vi "LVH5TGetLVType.vi"(7 "Don't use cache":bool, 8 "error in (no error)":errorcluster, 9 "Type":enum16{"File", "Memory"}(ring)=enum."Memory", 10 "Name":string, 11 "HDF5 Type Ref":T1) -> (0 "error out":errorcluster, 1 "Type String":i16[](array[numeric]) format="%.0x", 2 "Data Type":variant, 3 "HDF5 Type Ref out":T1, 4 "Description":string)   [LabVIEW 2017]
doc: "Creates a variant containg a LabVIEW datatype which corresponds to an HDF5 datatype."
uses:
  <vilib>/UPVI/lvhdf5/library.llb/HDF5 Ref.ctl
  <vilib>/UPVI/lvhdf5/datatype.llb/private/LVTypeElement.ctl
  <vilib>/Utility/VariantDataType/UnitInfo.ctl
  <vilib>/Utility/VariantDataType/UnitType.ctl
  <vilib>/UPVI/lvhdf5/error.llb/LVH5EMajorID.ctl
  <vilib>/UPVI/lvhdf5/error.llb/LVH5EMinorID.ctl
  <userlib>/_OpenG.lib/lvdata/lvdata.llb/Type Descriptor Enumeration__ogtk.ctl
  <vilib>/UPVI/lvhdf5/datatype.llb/H5T_sign_t.ctl
  <vilib>/UPVI/lvhdf5/datatype.llb/LVH5ClassID.ctl
  <vilib>/UPVI/lvhdf5/reference.llb/H5R Object Ref.ctl
  <vilib>/UPVI/lvhdf5/reference.llb/H5R Dataset Region Ref.ctl
  <vilib>/UPVI/lvhdf5/error.llb/H5Epush_enum_enum.vi
  <vilib>/Utility/VariantDataType/VariantType.lvlib
panel:
  # "LVHDF5 Toolkit\nCopyright (c) 2005-2013 by Jason D. Sommerville\nCopyright (c) 2014 by UPVI, LLC.\n\nThis use and distribution of this file is governed by the terms found in \nLICENSE.txt distributed with this toolkit and installed at\n <user.lib>\\_lvhdf5\\LICENSE.txt"
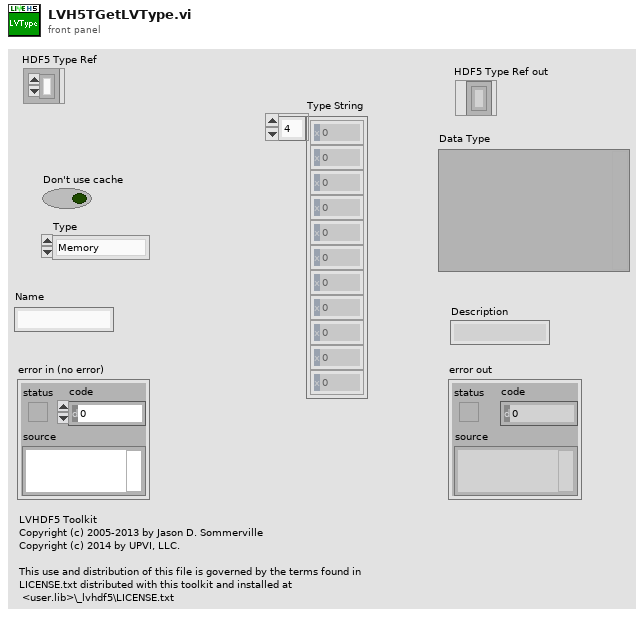
[diagram p1: front panel]
types:
  T1 = typedef "HDF5 Ref.ctl" = refnum<k1>
  T2 = enum16{"find by lvtype", "find by h5type", "index", "push", "pop", "delete last", "dequeue", "delete all"}
  T3 = typedef "LVTypeElement.ctl" = cluster{"Name":string, "TD":i16[], "Type Ref":T1, "Description":string, "Unit String":string, "Units":T4[], "Status":cluster{"MustCommit":bool, "IsCommitted":bool}}
  T4 = typedef "VariantType.lvlib/UnitInfo.ctl" = cluster{"UnitType":T5, "Exponent":i16}
  T5 = typedef "VariantType.lvlib/UnitType.ctl" = enum16{"Radians", "Steradians", "Seconds", "Meters", "Kilograms", "Amperes", "Kelvins", "Moles", "Candelas", "InvalidUnit"}
  T6 = typedef "LVH5EMinorID.ctl" = string
  T7 = typedef "LVH5EMajorID.ctl" = string
  T8 = typedef "Type Descriptor Enumeration__ogtk.ctl" = enum8{"<Null>", "I8", "I16", "I32", "I64", "U8", "U16", "U32", "U64", "SGL", "DBL", "EXT", "CSG", "CDB", "CXT", "0x0F", "0x10", "0x11", "0x12", "0x13", "0x14", "Enum U8", "Enum U16", "Enum U32", "Enum U64", "SGL PQ", "DBL PQ", "EXT PQ", "CSG PQ", "CDB PQ", "CXT PQ", "0x1F", "0x20", "Boolean", "0x22", "0x23", "0x24", "0x25", "0x26", "0x27", "0x28", "0x29", "0x2A", "0x2B", "0x2C", "0x2D", "0x2E", "0x2F", "String", "0x31", "Path", "Pict", "0x34", "0x35", "0x36", "DAQ", "0x38", "0x39", "0x3A", "0x3B", "0x3C", "0x3D", "0x3E", "0x3F", "Array", "0x41", "0x42", "0x43", "0x44", "0x45", "0x46", "0x47", "0x48", "0x49", "0x4A", "0x4B", "0x4C", "0x4D", "0x4E", "0x4F", "Cluster", "0x51", "0x52", "Variant", "Waveform", "0x55", "0x56", "0x57", "0x58", "0x59", "0x5A", "0x5B", "0x5C", "0x5D", "0x5E", "0x5F", "0x60", "0x61", "0x62", "0x63", "0x64", "0x65", "0x66", "0x67", "0x68", "0x69", "0x6A", "0x6B", "0x6C", "0x6D", "0x6E", "0x6F", "Refnum"}
  T9 = typedef "LVH5ClassID.ctl" = enum32{"H5T_IEEE_F32BE", "H5T_IEEE_F32LE", "H5T_IEEE_F64BE", "H5T_IEEE_F64LE", "H5T_STD_I8BE", "H5T_STD_I8LE", "H5T_STD_I16BE", "H5T_STD_I16LE", "H5T_STD_I32BE", "H5T_STD_I32LE", "H5T_STD_I64BE", "H5T_STD_I64LE", "H5T_STD_U8BE", "H5T_STD_U8LE", "H5T_STD_U16BE", "H5T_STD_U16LE", "H5T_STD_U32BE", "H5T_STD_U32LE", "H5T_STD_U64BE", "H5T_STD_U64LE", "H5T_STD_B8BE", "H5T_STD_B8LE", "H5T_STD_B16BE", "H5T_STD_B16LE", "H5T_STD_B32BE", "H5T_STD_B32LE", "H5T_STD_B64BE", "H5T_STD_B64LE", "H5T_STD_REF_OBJ", "H5T_STD_REF_DSETREG", "H5T_UNIX_D32BE", "H5T_UNIX_D32LE", "H5T_UNIX_D64BE", "H5T_UNIX_D64LE", "H5T_C_S1", "H5T_FORTRAN_S1", "H5T_INTEL_I8", "H5T_INTEL_I16", "H5T_INTEL_I32", "H5T_INTEL_I64", "H5T_INTEL_U8", "H5T_INTEL_U16", "H5T_INTEL_U32", "H5T_INTEL_U64", "H5T_INTEL_B8", "H5T_INTEL_B16", "H5T_INTEL_B32", "H5T_INTEL_B64", "H5T_INTEL_F32", "H5T_INTEL_F64", "H5T_ALPHA_I8", "H5T_ALPHA_I16", "H5T_ALPHA_I32", "H5T_ALPHA_I64", "H5T_ALPHA_U8", "H5T_ALPHA_U16", "H5T_ALPHA_U32", "H5T_ALPHA_U64", "H5T_ALPHA_B8", "H5T_ALPHA_B16", "H5T_ALPHA_B32", "H5T_ALPHA_B64", "H5T_ALPHA_F32", "H5T_ALPHA_F64", "H5T_MIPS_I8", "H5T_MIPS_I16", "H5T_MIPS_I32", "H5T_MIPS_I64", "H5T_MIPS_U8", "H5T_MIPS_U16", "H5T_MIPS_U32", "H5T_MIPS_U64", "H5T_MIPS_B8", "H5T_MIPS_B16", "H5T_MIPS_B32", "H5T_MIPS_B64", "H5T_MIPS_F32", "H5T_MIPS_F64", "H5T_NATIVE_CHAR", "H5T_NATIVE_SCHAR", "H5T_NATIVE_UCHAR", "H5T_NATIVE_SHORT", "H5T_NATIVE_USHORT", "H5T_NATIVE_INT", "H5T_NATIVE_UINT", "H5T_NATIVE_LONG", "H5T_NATIVE_ULONG", "H5T_NATIVE_LLONG", "H5T_NATIVE_ULLONG", "H5T_NATIVE_FLOAT", "H5T_NATIVE_DOUBLE", "H5T_NATIVE_LDOUBLE", "H5T_NATIVE_B8", "H5T_NATIVE_B16", "H5T_NATIVE_B32", "H5T_NATIVE_B64", "H5T_NATIVE_OPAQUE", "H5T_NATIVE_HADDR", "H5T_NATIVE_HSIZE", "H5T_NATIVE_HSSIZE", "H5T_NATIVE_HERR", "H5T_NATIVE_HBOOL", "H5T_NATIVE_INT8", "H5T_NATIVE_UINT8", "H5T_NATIVE_INT_LEAST8", "H5T_NATIVE_UINT_LEAST8", "H5T_NATIVE_INT_FAST8", "H5T_NATIVE_UINT_FAST8", "H5T_NATIVE_INT16", "H5T_NATIVE_UINT16", "H5T_NATIVE_INT_LEAST16", "H5T_NATIVE_UINT_LEAST16", "H5T_NATIVE_INT_FAST16", "H5T_NATIVE_UINT_FAST16", "H5T_NATIVE_INT32", "H5T_NATIVE_UINT32", "H5T_NATIVE_INT_LEAST32", "H5T_NATIVE_UINT_LEAST32", "H5T_NATIVE_INT_FAST32", "H5T_NATIVE_UINT_FAST32", "H5T_NATIVE_INT64", "H5T_NATIVE_UINT64", "H5T_NATIVE_INT_LEAST64", "H5T_NATIVE_UINT_LEAST64", "H5T_NATIVE_INT_FAST64"}
  T10 = typedef "H5T_sign_t.ctl" = i32
  T11 = typedef "H5R Object Ref.ctl" = refnum<k1>
  T12 = typedef "H5R Dataset Region Ref.ctl" = refnum<k1>
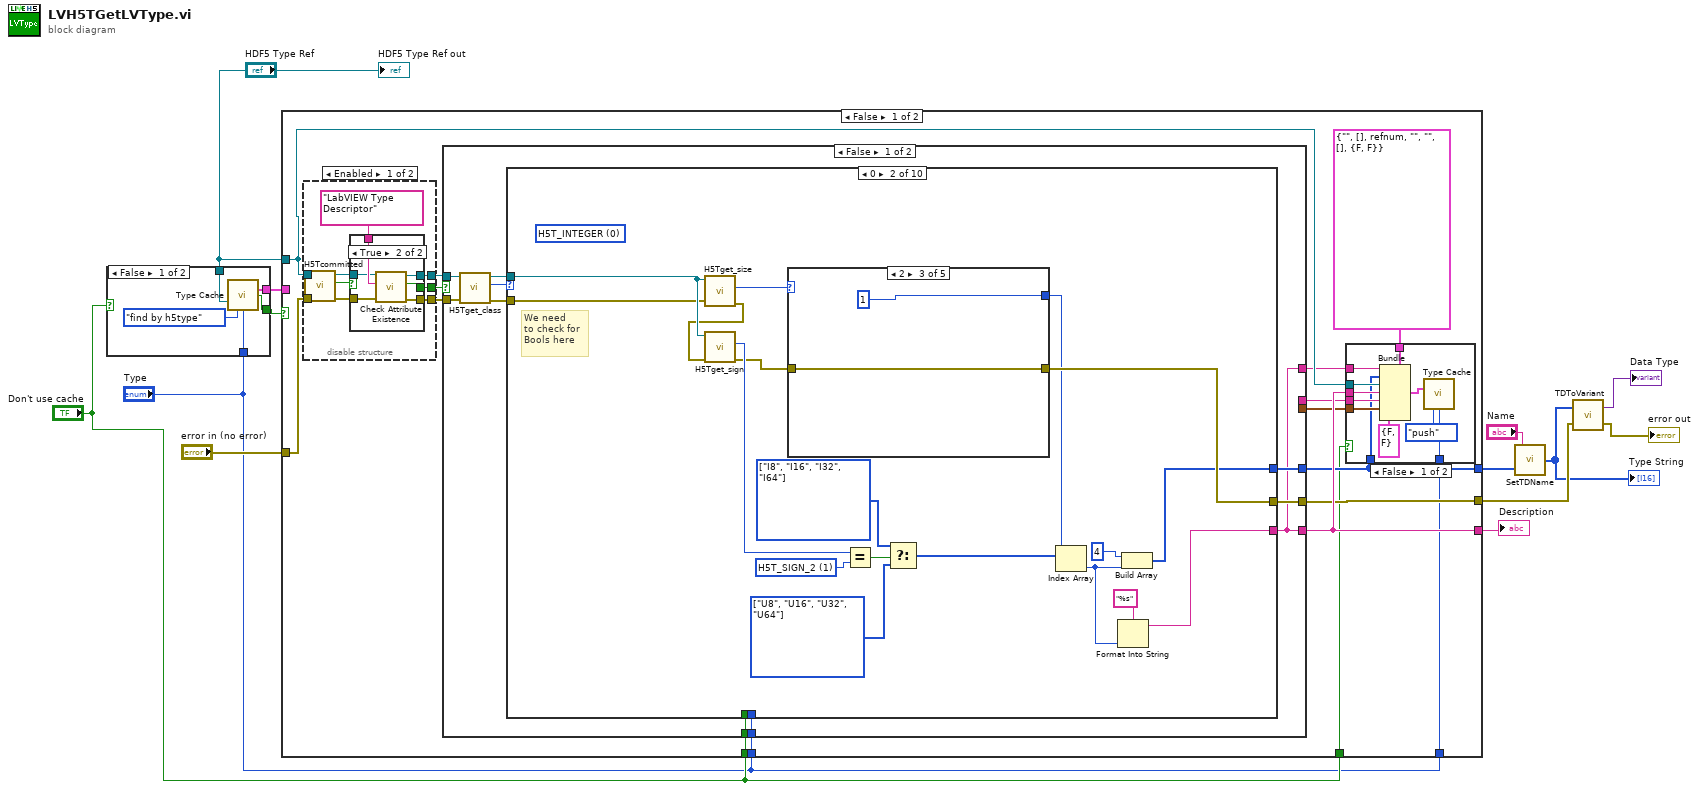
[diagram p0: block diagram]
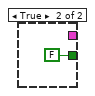
[diagram p2: hidden frame]
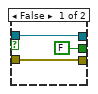
[diagram p4: hidden frame]
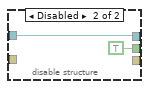
[diagram p5: hidden frame]
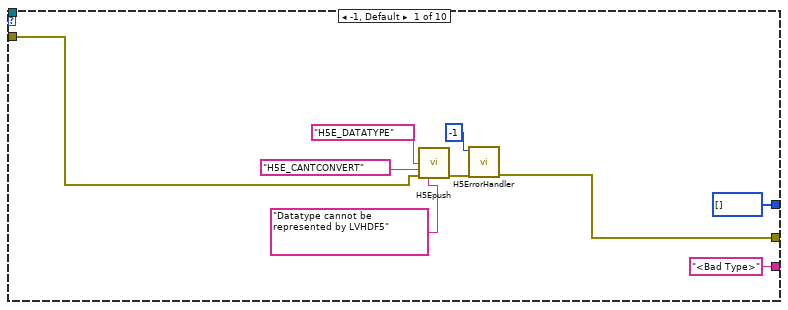
[diagram p6: hidden frame]
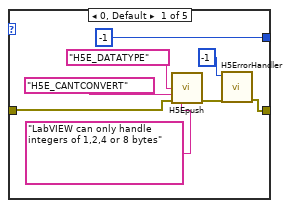
[diagram p7: hidden frame]
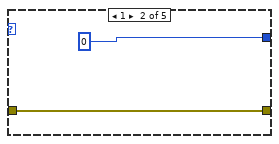
[diagram p8: hidden frame]
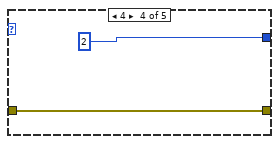
[diagram p9: hidden frame]
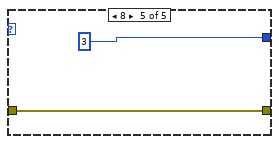
[diagram p10: hidden frame]
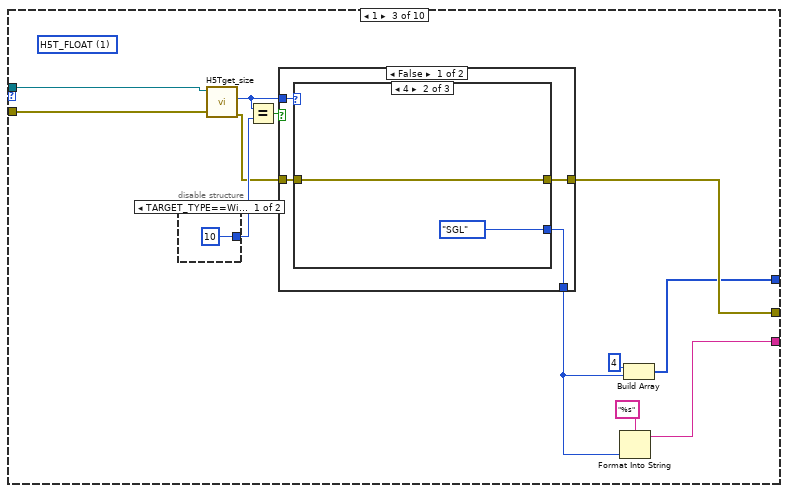
[diagram p11: hidden frame]
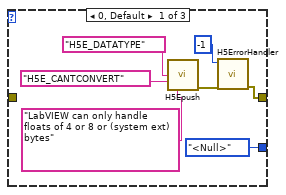
[diagram p12: hidden frame]
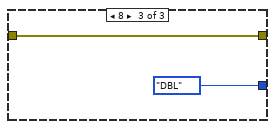
[diagram p13: hidden frame]
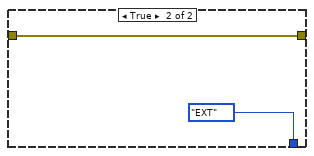
[diagram p14: hidden frame]
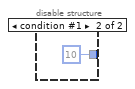
[diagram p15: hidden frame]
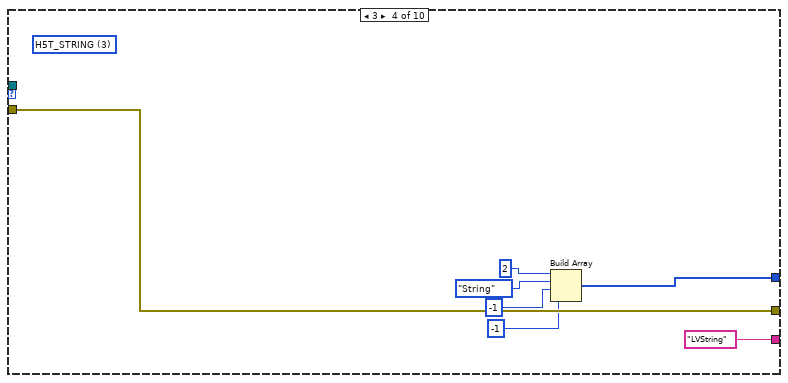
[diagram p16: hidden frame]
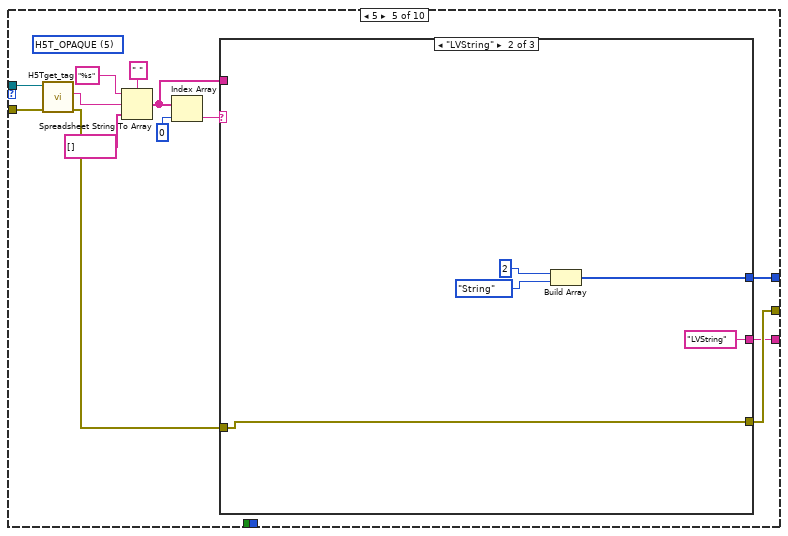
[diagram p17: hidden frame]
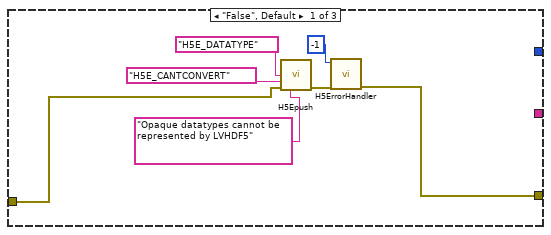
[diagram p18: hidden frame]
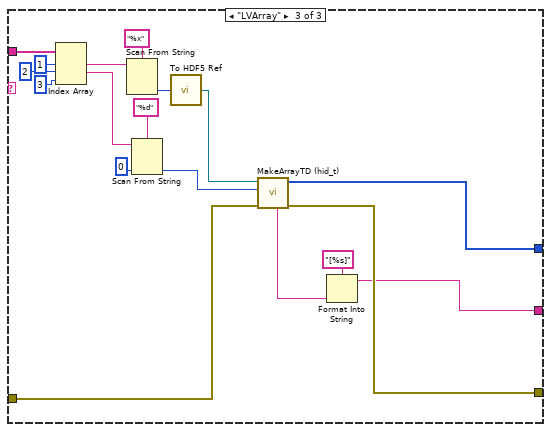
[diagram p19: hidden frame]
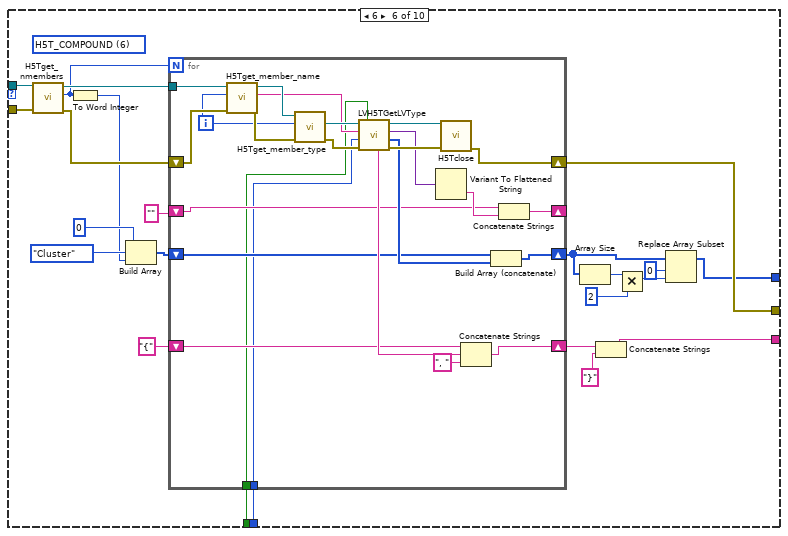
[diagram p20: hidden frame]
diagram:
  n1 = case shown="False" "Don't use cache" {
    tunnel: "HDF5 Type Ref" -> [w18 _]
    tunnel: [w17 _] -> w12
    tunnel: [w16 FALSE ("Found?")] -> w11
    tunnel: "Type" -> [w14 _]
    frame False {
      n2 = call <vilib>:"Type Cache.vi"("H5Type (for find)"=w18, "operation"=T2."find by h5type", "Type"=w14) -> ("LVTypeElement out"=w17:T3, "Found?"=w16:bool)  [unwired: 9 in, 2 out]
    }
    frame True {
    }
  }
  n3 = case shown="False" w11 {
    tunnel: "error in (no error)" -> [w32 w562]
    tunnel: [w24 w561] -> w8
    tunnel: "HDF5 Type Ref" -> [w30 _]
    tunnel: w12 -> [_ w564]
    tunnel: [w28 w563] -> w10
    tunnel: [w25 w562] -> w7
    tunnel: "Don't use cache" -> [w23 _]
    tunnel: "Type" -> [w22 _]
    tunnel: "Don't use cache" -> [w21 _]
    tunnel: "Type" -> [w20 _]
    frame False {
      n4 = disable-structure shown="Enabled" {
        disable-tunnel: [w55 _] -> w35
        disable-tunnel: [w54 TRUE ("Exists")] -> w34
        disable-tunnel: [w52 w66] -> w33
        disable-tunnel: w32 -> [w50 _]
        disable-tunnel: w30 -> [w47 w66]
        frame Enabled {
          n5 = call <vilib>:"H5Tcommitted.vi"("error in (no error)"=w50, "HDF5Type  Ref"=w47) -> ("error out"=w49:errorcluster, "Committed"=w48:bool, "HDF5 Type Ref out"=w51:T1)  [unwired: 5 in]
          n6 = case shown="True" w48 {
            tunnel: [w56 w64] -> w55
            tunnel: [FALSE ("Exists") w63] -> w54
            tunnel: "LabVIEW Type Descriptor" ("name") -> [_ w62]
            tunnel: [w58 w61] -> w52
            tunnel: w51 -> [w58 w60]
            tunnel: w49 -> [w56 w59]
            frame False {
            }
            frame True {
              n7 = call <vilib>:"Check Attribute Existence.vi"("error in (no error)"=w59, "name"=w62, "HDF5 Ref"=w60) -> ("error out"=w64:errorcluster, "Exists"=w63:bool, "HDF5 Ref out"=w61:T1)  [unwired: 4 in]
            }
          }
        }
        frame Disabled {
        }
      }
      n8 = case shown="False" w34 {
        tunnel: [w69 w552] -> w28
        tunnel: [w73 w560] -> w24
        tunnel: [w72 w557] -> w25
        tunnel: w33 -> [w71 w556]
        tunnel: w35 -> [w70 w555]
        tunnel: [w69 w547] -> w29
        tunnel: [_ w559] -> w27
        tunnel: [_ w558] -> w26
        tunnel: w21 -> [w68 _]
        tunnel: w20 -> [w67 _]
        frame False {
          n9 = call <vilib>:"H5Tget_class.vi"("error in (no error)"=w70, "HDF5 Type Ref"=w71) -> ("error out"=w74:errorcluster, "class"=w76:i32, "HDF5 Type Ref out"=w75:T1)  [unwired: 5 in]
          n10 = case shown="0" w76 {
            tunnel: w75 -> [_ w103 w131 _ w170 w223 w255 w300 w529 w544]
            tunnel: w74 -> [w79 w102 w130 w153 w169 w222 w258 w298 w528 w543]
            tunnel: [i16[] [] ("td") w100 w128 w157 w163 w219 w250 w296 w531 w546] -> w73
            tunnel: [w80 w101 w129 w153 w159 w220 w248 w295 w527 w542] -> w72
            tunnel: ["<Bad Type>" w99 w127 "LVString" w158 w221 w249 w294 w530 w545] -> w69
            tunnel: w68 -> [_ _ _ _ _ w201 _ _ w520 w533]
            tunnel: w67 -> [_ _ _ _ _ w202 _ _ w519 w532]
            frame -1, Default {
              n11 = call-poly <vilib>:"H5Epush.vi"("major_id"=T7 "H5E_DATATYPE", "minor_id"=T6 "H5E_CANTCONVERT", "error in (no error)"=w79, "msg"="Datatype cannot be represented by LVHDF5") -> ("error out"=w81:errorcluster)  [unwired: 10 in, 1 out]
              n12 = call <vilib>:"H5ErrorHandler.vi"("error in (no error)"=w81, "herr_t"=-1) -> ("error out"=w80:errorcluster)  [unwired: 3 in, 4 out]
            }
            frame 0 {
              w97 = T10 1 items=["H5T_SIGN_ERROR"=-1, "H5T_SIGN_NONE"=0, "H5T_SIGN_2"=1] ("Sign")
              w93 = T8[] [enum."U8", enum."U16", enum."U32", enum."U64"] items=["<Null>", "I8", "I16", "I32", "I64", "U8", "U16", "U32", "U64", "SGL", "DBL", "EXT", "CSG", "CDB", "CXT", "0x0F", "0x10", "0x11", "0x12", "0x13", "0x14", "Enum U8", "Enum U16", "Enum U32", "Enum U64", "SGL PQ", "DBL PQ", "EXT PQ", "CSG PQ", "CDB PQ", "CXT PQ", "0x1F", "0x20", "Boolean", "0x22", "0x23", "0x24", "0x25", "0x26", "0x27", "0x28", "0x29", "0x2A", "0x2B", "0x2C", "0x2D", "0x2E", "0x2F", "String", "0x31", "Path", "Pict", "0x34", "0x35", "0x36", "DAQ", "0x38", "0x39", "0x3A", "0x3B", "0x3C", "0x3D", "0x3E", "0x3F", "Array", "0x41", "0x42", "0x43", "0x44", "0x45", "0x46", "0x47", "0x48", "0x49", "0x4A", "0x4B", "0x4C", "0x4D", "0x4E", "0x4F", "Cluster", "0x51", "0x52", "Variant", "Waveform", "0x55", "0x56", "0x57", "0x58", "0x59", "0x5A", "0x5B", "0x5C", "0x5D", "0x5E", "0x5F", "0x60", "0x61", "0x62", "0x63", "0x64", "0x65", "0x66", "0x67", "0x68", "0x69", "0x6A", "0x6B", "0x6C", "0x6D", "0x6E", "0x6F", "Refnum"]
              w94 = T8[] [enum."I8", enum."I16", enum."I32", enum."I64"] items=["<Null>", "I8", "I16", "I32", "I64", "U8", "U16", "U32", "U64", "SGL", "DBL", "EXT", "CSG", "CDB", "CXT", "0x0F", "0x10", "0x11", "0x12", "0x13", "0x14", "Enum U8", "Enum U16", "Enum U32", "Enum U64", "SGL PQ", "DBL PQ", "EXT PQ", "CSG PQ", "CDB PQ", "CXT PQ", "0x1F", "0x20", "Boolean", "0x22", "0x23", "0x24", "0x25", "0x26", "0x27", "0x28", "0x29", "0x2A", "0x2B", "0x2C", "0x2D", "0x2E", "0x2F", "String", "0x31", "Path", "Pict", "0x34", "0x35", "0x36", "DAQ", "0x38", "0x39", "0x3A", "0x3B", "0x3C", "0x3D", "0x3E", "0x3F", "Array", "0x41", "0x42", "0x43", "0x44", "0x45", "0x46", "0x47", "0x48", "0x49", "0x4A", "0x4B", "0x4C", "0x4D", "0x4E", "0x4F", "Cluster", "0x51", "0x52", "Variant", "Waveform", "0x55", "0x56", "0x57", "0x58", "0x59", "0x5A", "0x5B", "0x5C", "0x5D", "0x5E", "0x5F", "0x60", "0x61", "0x62", "0x63", "0x64", "0x65", "0x66", "0x67", "0x68", "0x69", "0x6A", "0x6B", "0x6C", "0x6D", "0x6E", "0x6F", "Refnum"]
              (unwired) 0 items=["H5T_NO_CLASS"=-1, "H5T_INTEGER"=0, "H5T_FLOAT"=1, "H5T_TIME"=2, "H5T_STRING"=3, "H5T_BITFIELD"=4, "H5T_OPAQUE"=5, "H5T_COMPOUND"=6, "H5T_REFERENCE"=7, "H5T_ENUM"=8, "H5T_VLEN"=9, "H5T_ARRAY"=10] ("class")
              # "We need\nto check for\nBools here"
              n13 = call <vilib>:"H5Tget_size.vi"("error in (no error)"=w102, "HDF5 Type Ref"=w103) -> ("error out"=w98:errorcluster, "Size"=w86:u32)  [unwired: 5 in, 1 out]
              n14 = call <vilib>:"H5Tget_sign.vi"("error in (no error)"=w98, "HDF5 Ref"=w103) -> ("error out"=w90:errorcluster, "Sign"=w96:T10)  [unwired: 5 in, 1 out]
              n15 = case shown="2" w86 {
                tunnel: [-1 0 1 2 3] -> w91
                tunnel: w90 -> [w105 w112 w114 w116 w118]
                tunnel: [w104 w112 w114 w116 w118] -> w101
                frame 0, Default {
                  n16 = call-poly <vilib>:"H5Epush.vi"("major_id"=T7 "H5E_DATATYPE", "minor_id"=T6 "H5E_CANTCONVERT", "error in (no error)"=w105, "msg"="LabVIEW can only handle integers of 1,2,4 or 8 bytes") -> ("error out"=w106:errorcluster)  [unwired: 10 in, 1 out]
                  n17 = call <vilib>:"H5ErrorHandler.vi"("error in (no error)"=w106, "herr_t"=-1) -> ("error out"=w104:errorcluster)  [unwired: 3 in, 4 out]
                }
                frame 1 {
                }
                frame 2 {
                }
                frame 4 {
                }
                frame 8 {
                }
              }
              n18 = Equal?(x=w96, y=w97) -> (x = y?=w95:bool)
              n19 = Select(t=w94, s=w95, f=w93) -> (s? t:f=w92:T8[])
              n20 = Index Array(array=w92, index=w91) -> (element=w88:T8)
              n21 = Format Into String(format string="%s", w88) -> (resulting string=w99:string)  [unwired: 2 in, 1 out]
              n22 = Build Array(i16 4, w88) -> (w100:i16[])
            }
            frame 1 {
              (unwired) 1 items=["H5T_NO_CLASS"=-1, "H5T_INTEGER"=0, "H5T_FLOAT"=1, "H5T_TIME"=2, "H5T_STRING"=3, "H5T_BITFIELD"=4, "H5T_OPAQUE"=5, "H5T_COMPOUND"=6, "H5T_REFERENCE"=7, "H5T_ENUM"=8, "H5T_VLEN"=9, "H5T_ARRAY"=10] ("class")
              n23 = disable-structure shown="TARGET_TYPE==Windows||TARGET_TYPE==Unix" {
                disable-tunnel: [10 10] -> w124
                frame condition #0 (active) {
                }
                frame condition #1 {
                }
              }
              n24 = call <vilib>:"H5Tget_size.vi"("error in (no error)"=w130, "HDF5 Type Ref"=w131) -> ("error out"=w122:errorcluster, "Size"=w120:u32)  [unwired: 5 in, 1 out]
              n25 = Equal?(x=w120, y=w124) -> (x = y?=w123:bool)
              n26 = case shown="False" w123 {
                tunnel: [w135 Type_Descriptor_Enumeration__ogtk."EXT" ("Type Descriptor Enumeration")] -> w121
                tunnel: [w134 w147] -> w129
                tunnel: w120 -> [w133 _]
                tunnel: w122 -> [w132 w147]
                frame False {
                  n27 = case shown="4" w133 {
                    tunnel: [Type_Descriptor_Enumeration__ogtk."<Null>" ("Type Descriptor Enumeration") Type_Descriptor_Enumeration__ogtk."SGL" ("Type Descriptor Enumeration") Type_Descriptor_Enumeration__ogtk."DBL" ("Type Descriptor Enumeration")] -> w135
                    tunnel: [w137 w144 w146] -> w134
                    tunnel: w132 -> [_ w144 w146]
                    frame 0, Default {
                      n28 = call-poly <vilib>:"H5Epush.vi"("major_id"=T7 "H5E_DATATYPE", "minor_id"=T6 "H5E_CANTCONVERT", "msg"="LabVIEW can only handle floats of 4 or 8 or (system ext) bytes") -> ("error out"=w138:errorcluster)  [unwired: 11 in, 1 out]
                      n29 = call <vilib>:"H5ErrorHandler.vi"("error in (no error)"=w138, "herr_t"=-1) -> ("error out"=w137:errorcluster)  [unwired: 3 in, 4 out]
                    }
                    frame 4 {
                    }
                    frame 8 {
                    }
                  }
                }
                frame True {
                }
              }
              n30 = Format Into String(format string="%s", w121) -> (resulting string=w127:string)  [unwired: 2 in, 1 out]
              n31 = Build Array(i16 4, w121) -> (w128:i16[])
            }
            frame 3 {
              (unwired) 3 items=["H5T_NO_CLASS"=-1, "H5T_INTEGER"=0, "H5T_FLOAT"=1, "H5T_TIME"=2, "H5T_STRING"=3, "H5T_BITFIELD"=4, "H5T_OPAQUE"=5, "H5T_COMPOUND"=6, "H5T_REFERENCE"=7, "H5T_ENUM"=8, "H5T_VLEN"=9, "H5T_ARRAY"=10] ("class")
              n32 = Build Array(i16 2, Type_Descriptor_Enumeration__ogtk."String" ("Type Descriptor Enumeration"), i16 -1 ("element"), i16 -1 ("element")) -> (w157:i16[])
            }
            frame 5 {
              (unwired) 5 items=["H5T_NO_CLASS"=-1, "H5T_INTEGER"=0, "H5T_FLOAT"=1, "H5T_TIME"=2, "H5T_STRING"=3, "H5T_BITFIELD"=4, "H5T_OPAQUE"=5, "H5T_COMPOUND"=6, "H5T_REFERENCE"=7, "H5T_ENUM"=8, "H5T_VLEN"=9, "H5T_ARRAY"=10] ("class")
              n33 = call <vilib>:"H5Tget_tag.vi"("error in (no error)"=w169, "HDF5 Ref"=w170) -> ("error out"=w160:errorcluster, "Tag"=w166:string)  [unwired: 5 in, 1 out]
              n34 = Spreadsheet String To Array(delimiter (Tab)=" ", format string="%s", spreadsheet string=w166, array type (2D Dbl)=string[] []) -> (array=w162:string[])
              n35 = Index Array(array=w162, index=0) -> (element=w164:string)
              n36 = case shown="\"LVString\"" w164 {
                tunnel: [_ w180 w199] -> w163
                tunnel: w162 -> [_ _ w200]
                tunnel: w160 -> [w172 w178 w198]
                tunnel: [w171 w178 w197] -> w159
                tunnel: [_ "LVString" w196] -> w158
                frame "False", Default {
                  n37 = call-poly <vilib>:"H5Epush.vi"("major_id"=T7 "H5E_DATATYPE", "minor_id"=T6 "H5E_CANTCONVERT", "error in (no error)"=w172, "msg"="Opaque datatypes cannot be represented by LVHDF5") -> ("error out"=w173:errorcluster)  [unwired: 10 in, 1 out]
                  n38 = call <vilib>:"H5ErrorHandler.vi"("error in (no error)"=w173, "herr_t"=-1) -> ("error out"=w171:errorcluster)  [unwired: 3 in, 4 out]
                }
                frame "LVString" {
                  n39 = Build Array(i16 2, Type_Descriptor_Enumeration__ogtk."String" ("Type Descriptor Enumeration")) -> (w180:i16[])
                }
                frame "LVArray" {
                  n40 = Index Array(array=w200, index #1=1 ("index"), index #2=2 ("index"), index #3=3 ("index")) -> (element #1=w192:string, element #2=w187:string)  [unwired: 1 out]
                  n41 = Scan From String(format string="%x", input string=w192) -> (output 1=w190:u32)  [unwired: 3 in, 3 out]
                  n42 = Scan From String(format string="%d", input string=w187, default 1=u16 0 ("default value 1")) -> (output 1=w185:u16)  [unwired: 2 in, 3 out]
                  n43 = call <vilib>:"To HDF5 Ref.vi"("I32"=w190) -> ("HDF5 Ref"=w189:T1)
                  n44 = call <vilib>:"MakeArrayTD (hid_t).vi"("error in (no error)"=w198, "rank"=w185, "Element type_id"=w189) -> ("error out"=w197:errorcluster, "td"=w199:i16[], "Description"=w184:string)  [unwired: 5 in, 1 out]
                  n45 = Format Into String(format string="[%s]", w184) -> (resulting string=w196:string)  [unwired: 2 in, 1 out]
                }
              }
            }
            frame 6 {
              (unwired) 6 items=["H5T_NO_CLASS"=-1, "H5T_INTEGER"=0, "H5T_FLOAT"=1, "H5T_TIME"=2, "H5T_STRING"=3, "H5T_BITFIELD"=4, "H5T_OPAQUE"=5, "H5T_COMPOUND"=6, "H5T_REFERENCE"=7, "H5T_ENUM"=8, "H5T_VLEN"=9, "H5T_ARRAY"=10] ("class")
              n46 = call <vilib>:"H5Tget_nmembers.vi"("error in (no error)"=w222, "HDF5 Type Ref"=w223) -> ("error out"=w217:errorcluster, "nmembers"=w210:i32, "HDF5 Type Ref out"=w218:T1)  [unwired: 5 in]
              n47 = To Word Integer(number=w210) -> (16bit integer=w209:i16)
              n48 = Build Array(i16 0 ("element"), Type_Descriptor_Enumeration__ogtk."Cluster" ("Type Descriptor Enumeration"), w209) -> (w211:i16[])
              n49 = for {
                N: w210 -> [_]
                tunnel: w218 -> [w247]
                shift-right: [w233] -> w220
                shift-left: w217 -> [w246]
                shift-right: [w234] -> w215
                shift-left: "{" -> [w235]
                shift-right: [w230] -> w206
                shift-left: w211 -> [w231]
                shift-right: [w228] -> _
                shift-left: "" -> [w226]
                tunnel: w202 -> [w224]
                tunnel: w201 -> [w225]
                i -> [w243]
                n50 = call <vilib>:"H5Tget_member_name.vi"("error in (no error)"=w246, "Index"=w243, "HDF5 Compount Type Ref"=w247) -> ("error out"=w244:errorcluster, "name"=w241:string, "HDF5 Ref out"=w245:T1)  [unwired: 4 in]
                n51 = call <vilib>:"H5Tget_member_type.vi"("error in (no error)"=w244, "Member Number"=w243, "HDF5 Type Ref"=w245) -> ("error out"=w239:errorcluster, "HDF5 Member Type Ref"=w242:T1)  [unwired: 4 in, 1 out]
                n52 = call <vilib>:"LVH5TGetLVType.vi"("Don't use cache"=w225, "error in (no error)"=w239, "Type"=w224, "Name"=w241, "HDF5 Type Ref"=w242) -> ("error out"=w238:errorcluster, "Type String"=w232:i16[], "Data Type"=w229:variant, "HDF5 Type Ref out"=w240:T1, "Description"=w237:string)  [unwired: 2 in]
                n53 = Variant To Flattened String(Variant=w229) -> (data string=w227:string)  [unwired: 1 out]
                n54 = call <vilib>:"H5Tclose.vi"("error in (no error)"=w238, "HDF5 Datatype Ref"=w240) -> ("error out"=w233:errorcluster)  [unwired: 7 in]
                n55 = Concatenate Strings(w235, w237, ", " ("string")) -> (w234:string)
                n56 = Build Array (concatenate)(w231, w232) -> (w230:i16[])
                n57 = Concatenate Strings(w226, w227) -> (w228:string)
              }
              n58 = Array Size(array=w206) -> (size(s)=w208:i32)
              n59 = Concatenate Strings(w215, "}" ("string")) -> (w221:string)
              n60 = Multiply(x=w208, y=2) -> (x*y=w205:i32)
              n61 = Replace Array Subset(array=w206, new element=w205, index=i16 0) -> (w219:i16[])
            }
            frame 7 {
              (unwired) 7 items=["H5T_NO_CLASS"=-1, "H5T_INTEGER"=0, "H5T_FLOAT"=1, "H5T_TIME"=2, "H5T_STRING"=3, "H5T_BITFIELD"=4, "H5T_OPAQUE"=5, "H5T_COMPOUND"=6, "H5T_REFERENCE"=7, "H5T_ENUM"=8, "H5T_VLEN"=9, "H5T_ARRAY"=10] ("class")
              # "What type of ref is it?"
              n62 = call <vilib>:"LVH5TGetPredefinedType.vi"("error in"=w258, "H5 Standard Type"=LVH5ClassID."H5T_STD_REF_OBJ") -> ("error out"=w257:errorcluster, "HDF5 Ref"=w260:T1)  [unwired: 8 in]
              n63 = call <vilib>:"LVH5TGetPredefinedType.vi"("error in"=w257, "H5 Standard Type"=LVH5ClassID."H5T_STD_REF_DSETREG") -> ("error out"=w253:errorcluster, "HDF5 Ref"=w259:T1)  [unwired: 8 in]
              n64 = Build Array(w260, w259) -> (w256:T1[])
              n65 = for {
                tunnel: w256 -> [w288] mode=indexing
                tunnel: w255 -> [w287]
                shift-right: [w282] -> w252
                shift-left: -1 -> [w280]
                shift-right: [w284] -> w251
                shift-left: w253 -> [w286]
                i -> [w281]
                n66 = call <vilib>:"H5Tequal.vi"("error in (no error)"=w286, "HDF5 Ref 2"=w288, "HDF5 Ref"=w287) -> ("error out"=w283:errorcluster, "Equal"=w285:bool)  [unwired: 3 in, 2 out]
                n67 = case shown="True" w285 {
                  tunnel: [w290 w292] -> w284
                  tunnel: w283 -> [w290 w292]
                  tunnel: [w289 w291] -> w282
                  tunnel: w281 -> [_ w291]
                  tunnel: w280 -> [w289 _]
                  frame False {
                  }
                  frame True {
                  }
                }
              }
              n68 = case shown="0" w252 {
                tunnel: w251 -> [_ w271 w277]
                tunnel: [_ w273 w279] -> w250
                tunnel: ["<Bad Reference Type>" "H5R_OBJECT" "H5R_DSETREG"] -> w249
                tunnel: [w263 w271 w277] -> w248
                tunnel: [_ "\u0000\u0000\u0000\u0000" "\u0000\u0000\u0000\u0000"] -> _
                frame -1, Default {
                  n69 = call-poly <vilib>:"H5Epush.vi"("major_id"=T7 "H5E_DATATYPE", "minor_id"=T6 "H5E_CANTCONVERT", "msg"="Unrecognized HDF5 Reference Type") -> ("error out"=w264:errorcluster)  [unwired: 11 in, 1 out]
                  n70 = call <vilib>:"H5ErrorHandler.vi"("error in (no error)"=w264, "herr_t"=-1) -> ("error out"=w263:errorcluster)  [unwired: 3 in, 4 out]
                }
                frame 0 {
                  w274 = T11 refnum items=["H5R Object Handle"]
                  n71 = Variant To Flattened String(Variant=w274) -> (1:w273:i16[])  [unwired: 1 out]
                }
                frame 1 {
                  w276 = T12 refnum items=["H5R Dataset Region Handle"]
                  n72 = Variant To Flattened String(Variant=w276) -> (1:w279:i16[])  [unwired: 1 out]
                }
              }
            }
            frame 8 {
              (unwired) 8 items=["H5T_NO_CLASS"=-1, "H5T_INTEGER"=0, "H5T_FLOAT"=1, "H5T_TIME"=2, "H5T_STRING"=3, "H5T_BITFIELD"=4, "H5T_OPAQUE"=5, "H5T_COMPOUND"=6, "H5T_REFERENCE"=7, "H5T_ENUM"=8, "H5T_VLEN"=9, "H5T_ARRAY"=10] ("class")
              n73 = call <vilib>:"H5Tget_size.vi"("error in (no error)"=w298, "HDF5 Type Ref"=w300) -> ("error out"=w297:errorcluster, "Size"=w293:u32, "HDF5 Type Ref out"=w299:T1)  [unwired: 5 in]
              n74 = case shown="1" w293 {
                tunnel: w299 -> [_ w328 w381 w434 w487]
                tunnel: w297 -> [_ w309 w362 w415 w469]
                tunnel: [_ w310 w363 w416 w470] -> w296
                tunnel: [w301 w309 w362 w415 w469] -> w295
                tunnel: [_ "Enum U8" "Enum U16" "Enum U32" "Enum U64"] -> w294
                frame 0, Default {
                  n75 = call-poly <vilib>:"H5Epush.vi"("major_id"=T7 "H5E_DATATYPE", "minor_id"=T6 "H5E_CANTCONVERT", "msg"="Datatype cannot be represented by LVHDF5") -> ("error out"=w302:errorcluster)  [unwired: 11 in, 1 out]
                  n76 = call <vilib>:"H5ErrorHandler.vi"("error in (no error)"=w302, "herr_t"=-1) -> ("error out"=w301:errorcluster)  [unwired: 3 in, 4 out]
                }
                frame 1 {
                  n77 = while {
                    tunnel: w328 -> [w349]
                    tunnel: u8 255 -> [w345]
                    shift-right: [w338] -> w320
                    shift-left: u8[] [] -> [w339]
                    shift-right: [w335] -> w317
                    shift-left: i16 0 -> [w336]
                    i -> [w346]
                    stop <- w337 stop-if-true
                    # "Truncate"
                    n78 = To Unsigned Byte Integer(number=w346) -> (unsigned 8bit integer=w348:u8)
                    n79 = call <vilib>:"H5Tenum_nameof.vi"("Member Value"=w348, "HDF5 Type Ref"=w349) -> ("error out"=w347:errorcluster, "Member Name"=w342:string)  [unwired: 5 in, 1 out]
                    n80 = Greater Or Equal?(x=w346, y=w345) -> (x >= y?=w343:bool)
                    n81 = Unbundle By Name(w347) -> ("status"=w344:bool)
                    n82 = Or(x=w344, y=w343) -> (x .or. y?=w337:bool)
                    n83 = String Subset(string=w342, length (rest)=255 ("length (rest)")) -> (substring=w340:string)  [unwired: 1 in]
                    n84 = case shown="False" w337 {
                      tunnel: w340 -> [w357 _]
                      tunnel: w339 -> [w355 w359]
                      tunnel: [w352 w359] -> w338
                      tunnel: w336 -> [w351 w358]
                      tunnel: [w350 w358] -> w335
                      frame False {
                        n85 = String Length(string=w357) -> (length=w356:i32)
                        n86 = String To Byte Array(string=w357) -> (unsigned byte array=w353:u8[])
                        n87 = To Unsigned Byte Integer(number=w356) -> (unsigned 8bit integer=w354:u8)
                        n88 = Increment(x=w351) -> (x+1=w350:i16)
                        n89 = Build Array (concatenate)(w355, w354, w353) -> (w352:u8[])
                      }
                      frame True {
                      }
                    }
                  }
                  n90 = Array Size(array=w320) -> (size(s)=w324:i32)
                  n91 = Increment(x=w324) -> (x+1=w323:i32)
                  n92 = Quotient & Remainder(x=w323, y=2) -> (x-y*floor(x/y)=w321:i32, floor(x/y)=w319:i32)
                  n93 = case shown="0, Default" w321 {
                    tunnel: w320 -> [w332 w333]
                    tunnel: w319 -> [w330 w334]
                    tunnel: [w330 w334] -> _
                    tunnel: [w329 w333] -> w314
                    frame 0, Default {
                      # "Odd length array\nAdd one null"
                      n94 = Build Array (concatenate)(w332, u8 0) -> (w329:u8[])
                    }
                    frame 1 {
                      # "Even length array"
                    }
                  }
                  n95 = Array Size(array=w314) -> (size(s)=w313:i32)
                  n96 = Type Cast(type=i16[] [], x=w314) -> (*(type *) &x=w315:i16[])
                  n97 = Add(x=w313, y=6) -> (x+y=w311:i32)
                  n98 = To Word Integer(number=w311) -> (16bit integer=w307:i16)
                  n99 = Build Array (concatenate)(w307, Type_Descriptor_Enumeration__ogtk."Enum U8" ("Type Descriptor Enumeration"), w317, w315) -> (w310:i16[])
                }
                frame 2 {
                  n100 = while {
                    tunnel: w381 -> [w402]
                    tunnel: u16 65535 -> [w398]
                    shift-right: [w391] -> w373
                    shift-left: u8[] [] -> [w392]
                    shift-right: [w388] -> w370
                    shift-left: i16 0 -> [w389]
                    i -> [w399]
                    stop <- w390 stop-if-true
                    # "Truncate"
                    n101 = To Unsigned Word Integer(number=w399) -> (unsigned 16bit integer=w401:u16)
                    n102 = call <vilib>:"H5Tenum_nameof.vi"("Member Value"=w401, "HDF5 Type Ref"=w402) -> ("error out"=w400:errorcluster, "Member Name"=w395:string)  [unwired: 5 in, 1 out]
                    n103 = Greater Or Equal?(x=w399, y=w398) -> (x >= y?=w396:bool)
                    n104 = Unbundle By Name(w400) -> ("status"=w397:bool)
                    n105 = Or(x=w397, y=w396) -> (x .or. y?=w390:bool)
                    n106 = String Subset(string=w395, length (rest)=255 ("length (rest)")) -> (substring=w393:string)  [unwired: 1 in]
                    n107 = case shown="False" w390 {
                      tunnel: w393 -> [w410 _]
                      tunnel: w392 -> [w408 w412]
                      tunnel: [w405 w412] -> w391
                      tunnel: w389 -> [w404 w411]
                      tunnel: [w403 w411] -> w388
                      frame False {
                        n108 = String Length(string=w410) -> (length=w409:i32)
                        n109 = String To Byte Array(string=w410) -> (unsigned byte array=w406:u8[])
                        n110 = To Unsigned Byte Integer(number=w409) -> (unsigned 8bit integer=w407:u8)
                        n111 = Increment(x=w404) -> (x+1=w403:i16)
                        n112 = Build Array (concatenate)(w408, w407, w406) -> (w405:u8[])
                      }
                      frame True {
                      }
                    }
                  }
                  n113 = Array Size(array=w373) -> (size(s)=w377:i32)
                  n114 = Increment(x=w377) -> (x+1=w376:i32)
                  n115 = Quotient & Remainder(x=w376, y=2) -> (x-y*floor(x/y)=w374:i32, floor(x/y)=w372:i32)
                  n116 = case shown="0, Default" w374 {
                    tunnel: w373 -> [w385 w386]
                    tunnel: w372 -> [w383 w387]
                    tunnel: [w383 w387] -> _
                    tunnel: [w382 w386] -> w367
                    frame 0, Default {
                      # "Odd length array\nAdd one null"
                      n117 = Build Array (concatenate)(w385, u8 0) -> (w382:u8[])
                    }
                    frame 1 {
                      # "Even length array"
                    }
                  }
                  n118 = Array Size(array=w367) -> (size(s)=w366:i32)
                  n119 = Type Cast(type=i16[] [], x=w367) -> (*(type *) &x=w368:i16[])
                  n120 = Add(x=w366, y=6) -> (x+y=w364:i32)
                  n121 = To Word Integer(number=w364) -> (16bit integer=w360:i16)
                  n122 = Build Array (concatenate)(w360, Type_Descriptor_Enumeration__ogtk."Enum U16" ("Type Descriptor Enumeration"), w370, w368) -> (w363:i16[])
                }
                frame 4 {
                  # "i is i32"
                  n123 = while {
                    tunnel: w434 -> [w455]
                    tunnel: u32 2147483647 -> [w451]
                    shift-right: [w444] -> w426
                    shift-left: u8[] [] -> [w445]
                    shift-right: [w441] -> w423
                    shift-left: i16 0 -> [w442]
                    i -> [w452]
                    stop <- w443 stop-if-true
                    # "Truncate"
                    n124 = To Unsigned Long Integer(number=w452) -> (unsigned 32bit integer=w454:u32)
                    n125 = call <vilib>:"H5Tenum_nameof.vi"("Member Value"=w454, "HDF5 Type Ref"=w455) -> ("error out"=w453:errorcluster, "Member Name"=w448:string)  [unwired: 5 in, 1 out]
                    n126 = Greater Or Equal?(x=w452, y=w451) -> (x >= y?=w449:bool)
                    n127 = Unbundle By Name(w453) -> ("status"=w450:bool)
                    n128 = Or(x=w450, y=w449) -> (x .or. y?=w443:bool)
                    n129 = String Subset(string=w448, length (rest)=255 ("length (rest)")) -> (substring=w446:string)  [unwired: 1 in]
                    n130 = case shown="False" w443 {
                      tunnel: w446 -> [w463 _]
                      tunnel: w445 -> [w461 w465]
                      tunnel: [w458 w465] -> w444
                      tunnel: w442 -> [w457 w464]
                      tunnel: [w456 w464] -> w441
                      frame False {
                        n131 = String Length(string=w463) -> (length=w462:i32)
                        n132 = String To Byte Array(string=w463) -> (unsigned byte array=w459:u8[])
                        n133 = To Unsigned Byte Integer(number=w462) -> (unsigned 8bit integer=w460:u8)
                        n134 = Increment(x=w457) -> (x+1=w456:i16)
                        n135 = Build Array (concatenate)(w461, w460, w459) -> (w458:u8[])
                      }
                      frame True {
                      }
                    }
                  }
                  n136 = Array Size(array=w426) -> (size(s)=w430:i32)
                  n137 = Increment(x=w430) -> (x+1=w429:i32)
                  n138 = Quotient & Remainder(x=w429, y=2) -> (x-y*floor(x/y)=w427:i32, floor(x/y)=w425:i32)
                  n139 = case shown="0, Default" w427 {
                    tunnel: w426 -> [w438 w439]
                    tunnel: w425 -> [w436 w440]
                    tunnel: [w436 w440] -> _
                    tunnel: [w435 w439] -> w420
                    frame 0, Default {
                      # "Odd length array\nAdd one null"
                      n140 = Build Array (concatenate)(w438, u8 0) -> (w435:u8[])
                    }
                    frame 1 {
                      # "Even length array"
                    }
                  }
                  n141 = Array Size(array=w420) -> (size(s)=w419:i32)
                  n142 = Type Cast(type=i16[] [], x=w420) -> (*(type *) &x=w421:i16[])
                  n143 = Add(x=w419, y=6) -> (x+y=w417:i32)
                  n144 = To Word Integer(number=w417) -> (16bit integer=w413:i16)
                  n145 = Build Array (concatenate)(w413, Type_Descriptor_Enumeration__ogtk."Enum U32" ("Type Descriptor Enumeration"), w423, w421) -> (w416:i16[])
                }
                frame 8 {
                  # "i is i32"
                  n146 = while {
                    tunnel: w487 -> [w508]
                    tunnel: u64 2147483647 -> [w504]
                    shift-right: [w497] -> w479
                    shift-left: u8[] [] -> [w498]
                    shift-right: [w494] -> w476
                    shift-left: i16 0 -> [w495]
                    i -> [w505]
                    stop <- w496 stop-if-true
                    # "Truncate"
                    n147 = To Unsigned Quad Integer(1:w505) -> (0:w507:u64)
                    n148 = call <vilib>:"H5Tenum_nameof.vi"("Member Value"=w507, "HDF5 Type Ref"=w508) -> ("error out"=w506:errorcluster, "Member Name"=w501:string)  [unwired: 5 in, 1 out]
                    n149 = Greater Or Equal?(x=w505, y=w504) -> (x >= y?=w502:bool)
                    n150 = Unbundle By Name(w506) -> ("status"=w503:bool)
                    n151 = Or(x=w503, y=w502) -> (x .or. y?=w496:bool)
                    n152 = String Subset(string=w501, length (rest)=255 ("length (rest)")) -> (substring=w499:string)  [unwired: 1 in]
                    n153 = case shown="False" w496 {
                      tunnel: w499 -> [w516 _]
                      tunnel: w498 -> [w514 w518]
                      tunnel: [w511 w518] -> w497
                      tunnel: w495 -> [w510 w517]
                      tunnel: [w509 w517] -> w494
                      frame False {
                        n154 = String Length(string=w516) -> (length=w515:i32)
                        n155 = String To Byte Array(string=w516) -> (unsigned byte array=w512:u8[])
                        n156 = To Unsigned Byte Integer(number=w515) -> (unsigned 8bit integer=w513:u8)
                        n157 = Increment(x=w510) -> (x+1=w509:i16)
                        n158 = Build Array (concatenate)(w514, w513, w512) -> (w511:u8[])
                      }
                      frame True {
                      }
                    }
                  }
                  n159 = Array Size(array=w479) -> (size(s)=w483:i32)
                  n160 = Increment(x=w483) -> (x+1=w482:i32)
                  n161 = Quotient & Remainder(x=w482, y=2) -> (x-y*floor(x/y)=w480:i32, floor(x/y)=w478:i32)
                  n162 = case shown="0, Default" w480 {
                    tunnel: w479 -> [w491 w492]
                    tunnel: w478 -> [w489 w493]
                    tunnel: [w489 w493] -> _
                    tunnel: [w488 w492] -> w473
                    frame 0, Default {
                      # "Odd length array\nAdd one null"
                      n163 = Build Array (concatenate)(w491, u8 0) -> (w488:u8[])
                    }
                    frame 1 {
                      # "Even length array"
                    }
                  }
                  n164 = Array Size(array=w473) -> (size(s)=w472:i32)
                  n165 = Type Cast(type=i16[] [], x=w473) -> (*(type *) &x=w474:i16[])
                  n166 = Add(x=w472, y=6) -> (x+y=w467:i32)
                  n167 = To Word Integer(number=w467) -> (16bit integer=w466:i16)
                  n168 = Build Array (concatenate)(w466, Type_Descriptor_Enumeration__ogtk."Enum U64" ("Type Descriptor Enumeration"), w476, w474) -> (w470:i16[])
                }
              }
            }
            frame 9 {
              (unwired) 9 items=["H5T_NO_CLASS"=-1, "H5T_INTEGER"=0, "H5T_FLOAT"=1, "H5T_TIME"=2, "H5T_STRING"=3, "H5T_BITFIELD"=4, "H5T_OPAQUE"=5, "H5T_COMPOUND"=6, "H5T_REFERENCE"=7, "H5T_ENUM"=8, "H5T_VLEN"=9, "H5T_ARRAY"=10] ("class")
              n169 = call <vilib>:"H5Tget_super.vi"("error in (no error)"=w528, "HDF5 Type Ref"=w529) -> ("error out"=w524:errorcluster, "HDF5 Super Type Ref"=w522:T1)  [unwired: 5 in, 1 out]
              n170 = call <vilib>:"MakeArrayTD (hid_t).vi"("Use Cache"=w520, "error in (no error)"=w524, "Type"=w519, "rank"=u16 1, "Element type_id"=w522) -> ("error out"=w523:errorcluster, "td"=w531:i16[], "Description"=w526:string)  [unwired: 3 in, 1 out]
              n171 = call <vilib>:"H5Tclose.vi"("error in (no error)"=w523, "HDF5 Datatype Ref"=w522) -> ("error out"=w527:errorcluster)  [unwired: 7 in]
              n172 = Format Into String(format string="[%s]", w526) -> (resulting string=w530:string)  [unwired: 2 in, 1 out]
            }
            frame 10 {
              (unwired) 10 items=["H5T_NO_CLASS"=-1, "H5T_INTEGER"=0, "H5T_FLOAT"=1, "H5T_TIME"=2, "H5T_STRING"=3, "H5T_BITFIELD"=4, "H5T_OPAQUE"=5, "H5T_COMPOUND"=6, "H5T_REFERENCE"=7, "H5T_ENUM"=8, "H5T_VLEN"=9, "H5T_ARRAY"=10] ("class")
              n173 = call <vilib>:"H5Tget_super.vi"("error in (no error)"=w543, "HDF5 Type Ref"=w544) -> ("error out"=w537:errorcluster, "HDF5 Super Type Ref"=w538:T1, "HDF5 Type Ref out"=w536:T1)  [unwired: 5 in]
              n174 = call <vilib>:"H5Tget_array_ndims.vi"("error in (no error)"=w537, "HDF5 Type Ref"=w536) -> ("error out"=w535:errorcluster, "Rank"=w534:i32)  [unwired: 5 in, 1 out]
              n175 = call <vilib>:"MakeArrayTD (hid_t).vi"("Use Cache"=w533, "error in (no error)"=w535, "Type"=w532, "rank"=w534, "Element type_id"=w538) -> ("error out"=w539:errorcluster, "td"=w546:i16[], "Description"=w541:string)  [unwired: 3 in, 1 out]
              n176 = call <vilib>:"H5Tclose.vi"("error in (no error)"=w539, "HDF5 Datatype Ref"=w538) -> ("error out"=w542:errorcluster)  [unwired: 7 in]
              n177 = Format Into String(format string="[%s]", w541) -> (resulting string=w545:string)  [unwired: 2 in, 1 out]
            }
          }
        }
        frame True {
          n178 = call <vilib>:"H5Iget_name.vi"("error in (no error)"=w555, "HDF5 Ref"=w556) -> ("error out"=w553:errorcluster, "Name"=w551:string, "HDF5 Ref out"=w554:T1)  [unwired: 4 in, 1 out]
          n179 = Reverse String(1:w551) -> (0:w550:string)
          n180 = call <vilib>:"Read LV Type Attrs.vi"("error in (no error)"=w553, "LVType Ref"=w554) -> ("error out"=w557:errorcluster, "Type Descriptor"=w560:i16[], "Type Name"=w552:string, "Unit String"=w559:string, "Units"=w558:T4[])  [unwired: 4 in, 1 out]
          n181 = Search/Split String(string=w550, search string/char (-)="/") -> (substring before match=w548:string)  [unwired: 1 in, 2 out]
          n182 = Reverse String(1:w548) -> (0:w547:string)
        }
      }
      n183 = case shown="False" w23 {
        tunnel: T3 {"Name"="", "TD"=[], "Type Ref"=refnum, "Description"="", "Unit String"="", "Units"=[], "Status"={"MustCommit"=FALSE, "IsCommitted"=FALSE}} ("LVTypeElement in") -> [w46 _]
        tunnel: w30 -> [w45 _]
        tunnel: w29 -> [w44 _]
        tunnel: w28 -> [w43 _]
        tunnel: w27 -> [w42 _]
        tunnel: w26 -> [w41 _]
        tunnel: w24 -> [w37 _]
        tunnel: w22 -> [w36 _]
        frame False {
          n184 = Bundle(cluster=w46, "Name"=w44, "TD"=w37, "Type Ref"=w45, "Description"=w43, "Unit String"=w42, "Units"=w41, "Status"=cluster{"MustCommit":bool, "IsCommitted":bool} {"MustCommit"=FALSE, "IsCommitted"=FALSE}) -> (w39:T3)
          n185 = call <vilib>:"Type Cache.vi"("LVTypeElement in"=w39, "operation"=T2."push", "Type"=w36) -> ()  [unwired: 9 in, 4 out]
        }
        frame True {
        }
      }
    }
    frame True {
      n186 = Unbundle By Name(w564) -> ("TD"=w561:i16[], "Description"=w563:string)
    }
  }
  "Description" <- w10
  n187 = call <vilib>:"SetTDName.vi"("Type Descriptor in"=w8, "Data Name"="Name") -> ("Type Descriptor out"=w5:i16[])
  "Type String" <- w5
  n188 = call <vilib>:"TDToVariant.vi"("error in (no error)"=w7, "Type Descriptor"=w5) -> ("error out"=→"error out":errorcluster, "Default Data"=→"Data Type":variant)
  "HDF5 Type Ref out" <- "HDF5 Type Ref"
